vi "joystick commands.vi"(11 "input cluster":T1) -> (3 "CTR to CMNDS":T2)   [LabVIEW 2014]
uses:
  Commands.ctl
  Controls.ctl
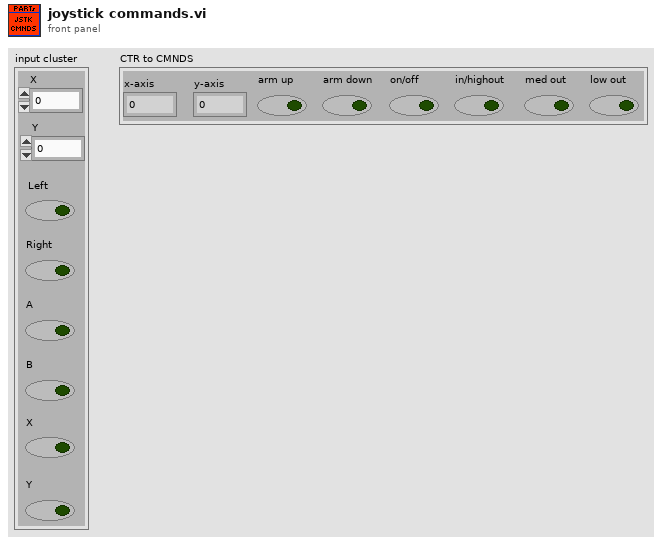
[diagram p1: front panel]
types:
  T1 = typedef "Controls.ctl" = cluster{"X":dbl, "Y":dbl, "Left":bool, "Right":bool, "A":bool, "B":bool, "X":bool, "Y":bool}
  T2 = typedef "Commands.ctl" = cluster{"x-axis":dbl, "y-axis":dbl, "arm up":bool, "arm down":bool, "on/off":bool, "in/highout":bool, "med out":bool, "low out":bool}
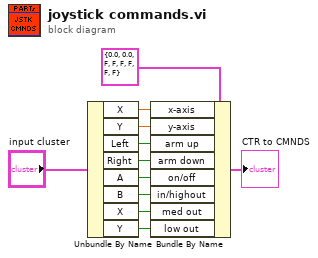
[diagram p0: block diagram]
diagram:
  n1 = Unbundle By Name("input cluster") -> ("X"=w2:dbl, "Y"=w3:dbl, "Left"=w4:bool, "Right"=w5:bool, "A"=w6:bool, "B"=w7:bool, "X"=w8:bool, "Y"=w9:bool)
  n2 = Bundle By Name(cluster=T2 {"x-axis"=0.0, "y-axis"=0.0, "arm up"=FALSE, "arm down"=FALSE, "on/off"=FALSE, "in/highout"=FALSE, "med out"=FALSE, "low out"=FALSE} ("CTR to CMNDS"), "x-axis"=w2, "y-axis"=w3, "arm up"=w4, "arm down"=w5, "on/off"=w6, "in/highout"=w7, "med out"=w8, "low out"=w9) -> (→"CTR to CMNDS":T2)
